vi "Write Controller Address.vi"(8 "error in (no error)":errorcluster, 10 "Controller":T1, 11 "Controller Message in":refnum<class "Controller Message.lvclass">) -> (0 "error out":errorcluster, 3 "Controller Message out":refnum<class "Controller Message.lvclass">)   [LabVIEW 2015, in "RDS Child Messages.lvlib" / "Controller Message.lvclass"]
uses:
  Controller Message.lvclass
  Actors/RDS Controller Actor/RDS Controller Actor/Controller.ctl
  Controller Message.lvclass/Controller Message.ctl
  Actors/RDS Controller Actor/RDS Controller Actor/RDS Controller Actor.lvlib
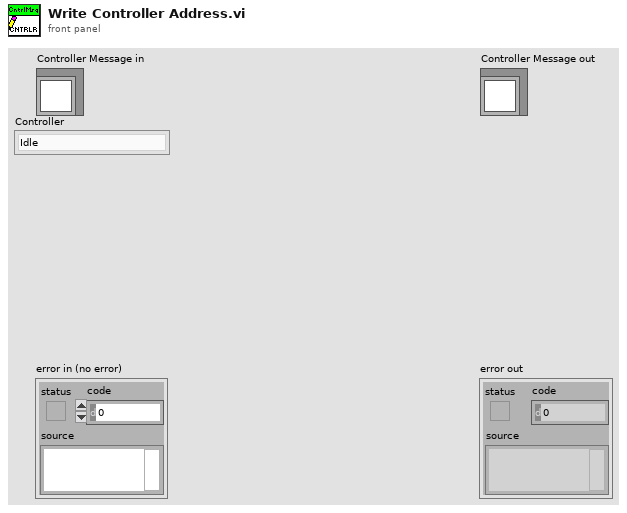
[diagram p1: front panel]
types:
  T1 = typedef "RDS Controller Actor.lvlib/Controller.ctl" = enum16{"Idle", "Local Remote Control", "Shore Remote Control", "Mission Control"}
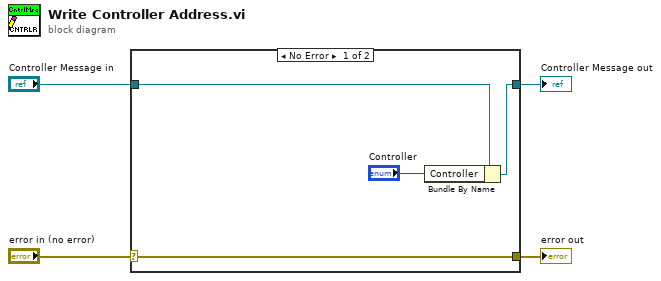
[diagram p0: block diagram]
diagram:
  n1 = case shown="No Error" "error in (no error)" {
    selector: "error in (no error)" -> [w8 w9]
    tunnel: [w8 w9] -> w3
    tunnel: [w6 w10] -> w1
    tunnel: "Controller Message in" -> [w7 w10]
    frame No Error {
      n2 = Bundle By Name(cluster=w7, "Controller"="Controller") -> (w6:refnum<class "Controller Message.lvclass">)
    }
    frame Error {
    }
  }
  "error out" <- w3
  "Controller Message out" <- w1
